vi "Read_Camram_Example.vi"() -> ()   [LabVIEW 2019]
uses:
  camera/Camera.lvclass
  <vilib>/picture/picture.llb/Draw True-Color Pixmap.vi
  <vilib>/picture/picture.llb/Draw 8-Bit Pixmap.vi
panel:
  out "colormap(U8)":u32[](array[numeric])
  out "Image(U16)":u16[][](graph)
  in  "Zoom [%]":i32(slide)=26 min=10 max=200 step=5 scale=10.0..200.0
  out "Image":picture
  out "rawImage":u16[][](array[numeric])
  in  "data_format":T1(ring)=enum."Mono16"
  in  "Image Index":u32 max=1084
  out "Recorded Images":u32
  in  "Quit":bool
  in  "roiY1":u64=2 min=2 max=1440 step=1
  in  "roiX1":u64=2 min=2 max=1920 step=1
  in  "roiY0":u64=1 min=1 max=1439 step=1
  in  "roiX0":u64=1 min=1 max=1919 step=1
  out "Image Height":u16
  out "Image Width":u16
  in  "segment":u16=3 caption="Segment" min=1 max=4
  out "Error":errorcluster {"code" format="%x"}
  # "This example shows for cameras with internal memory how to read images from ram, already available from a previous record\nIt is a good starting point for writing own applications.\nBut it will not be fail save, i.e. doesnt react on errors, just handles them forward to the end\n\nUsage:\nSelect the segment you want to read from before you start the program. \nThis segment must already contain images, otherwise the read will fail\nOnce started, the camera class will be initialized and images will be recorded automatically.\nWhen acquisition has finished you can address the images and set a certain roi \nTo finish the program click on quit application, this will force fan exit of the camera class"
  # "pco.labview"
  # "Camera Setup"
  # "Recording Control"
  # "Parameters for image readout"
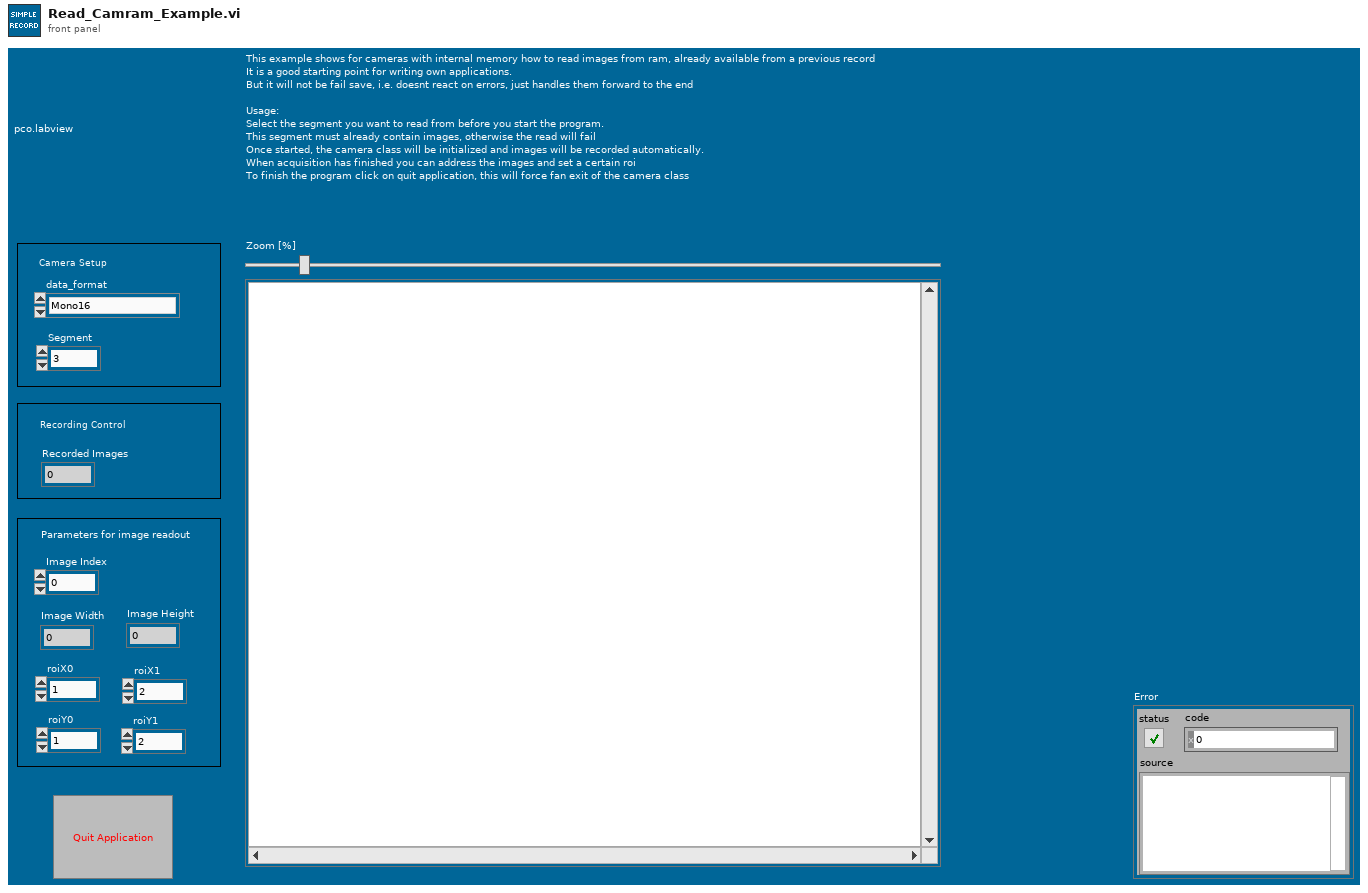
[diagram p1: front panel]
types:
  T1 = enum16{"Undefined", "Mono8", "Mono16", "BGRA8", "RGBA8", "BGRA16", "RGBA16", "CompressedMono8"}
  T2 = enum8{"Enabled", "Disabled", "Disabled and Grayed Out"}
  T3 = typedef "Camera.lvclass/binning.ctl" = cluster{"vert":u16, "horz":u16, "mode":u16}
  T4 = cluster{"exposure_time_s":dbl, "delay_time_s":dbl, "roi":cluster{"x0":u64, "y0":u64, "x1":u64, "y1":u64}, "timestamp_mode":u16, "pixelrate":u32, "conversion_factor":sgl, "trigger_mode":u16, "acquire_mode":u16, "acquire_sequence_number":u32, "metadata_mode":u16, "noisefilter_mode":u16, "pixel_format":u32, "binning":T3, "auto_exposure":cluster{"region":u16, "min_exposure_s":dbl, "max_exposure_s":dbl}}
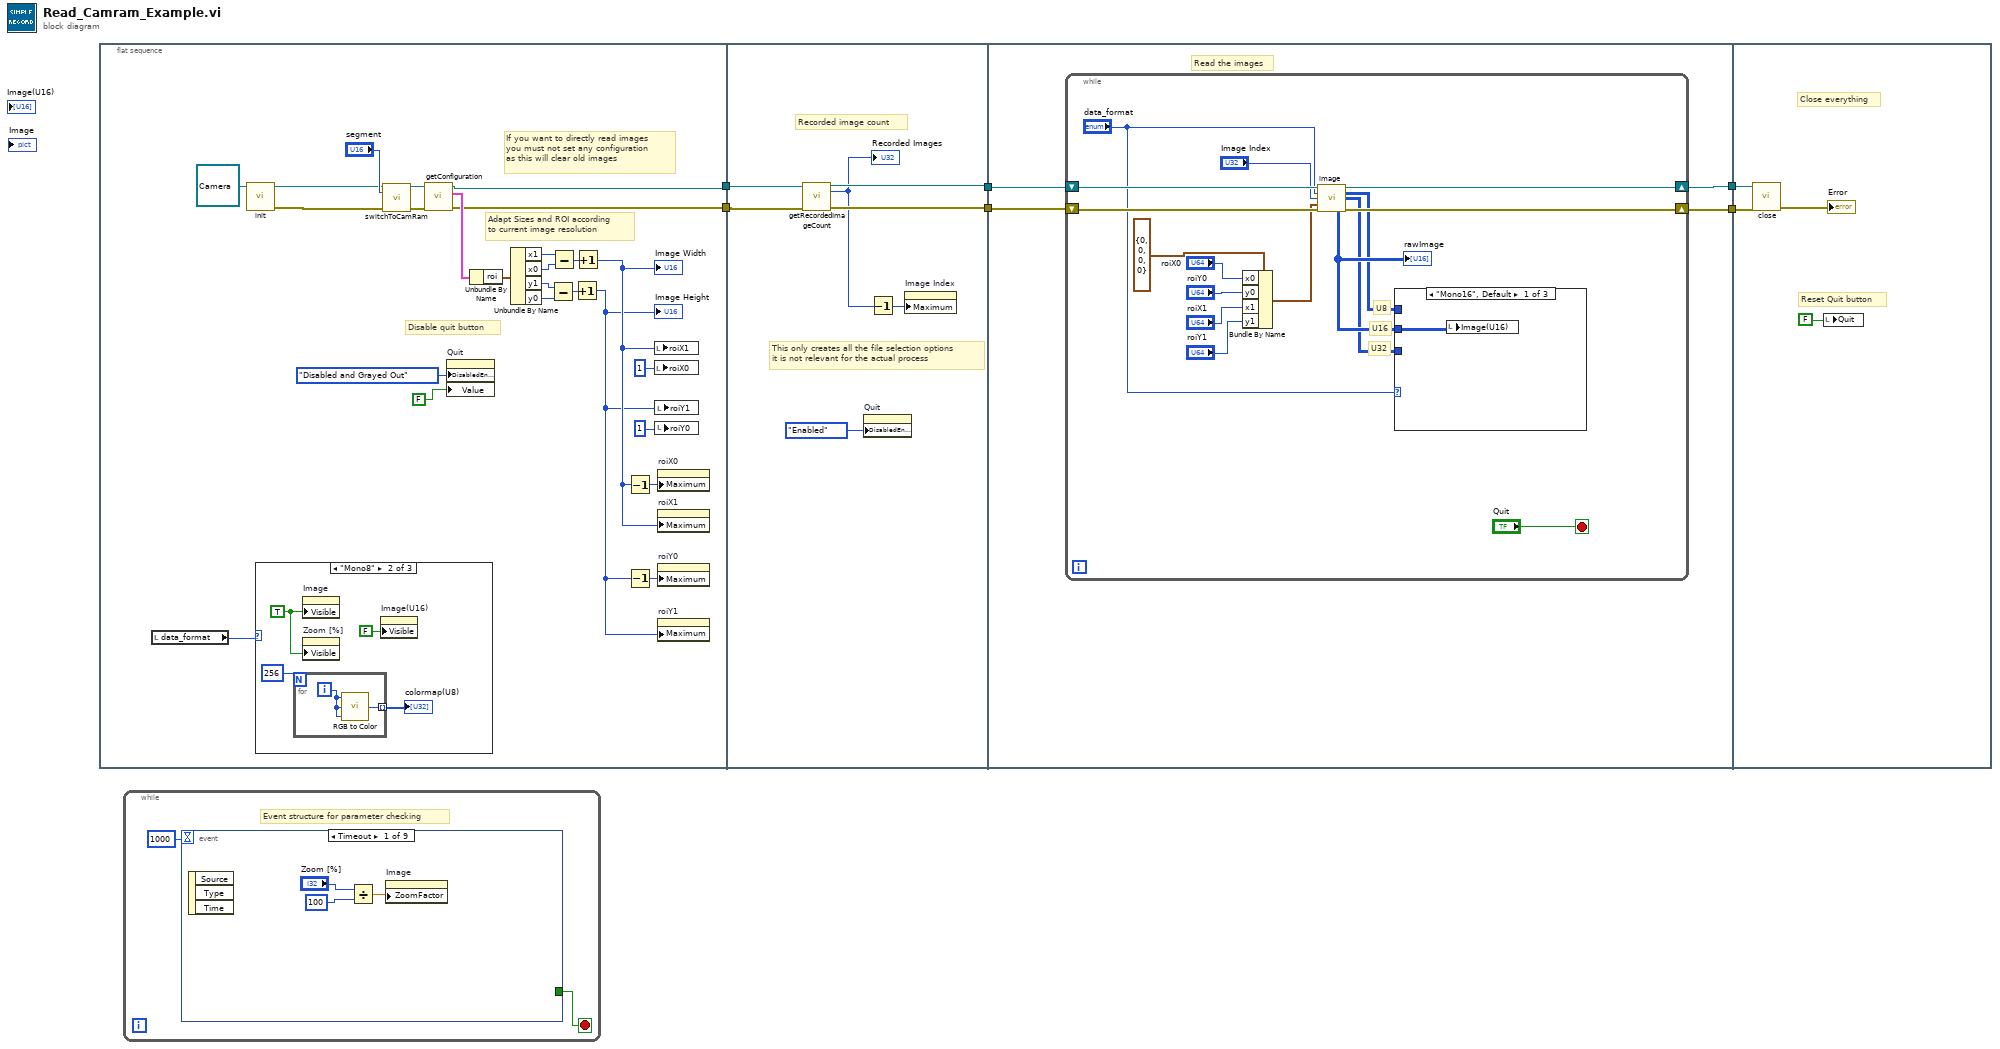
[diagram p0: block diagram]
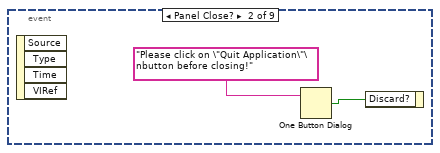
[diagram p2: hidden frame]
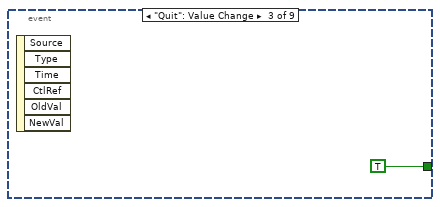
[diagram p3: hidden frame]
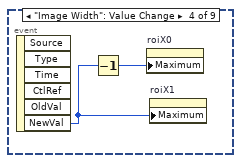
[diagram p4: hidden frame]
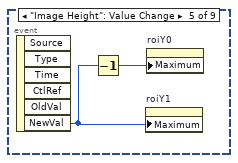
[diagram p5: hidden frame]
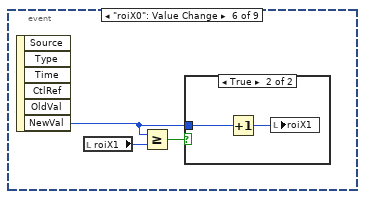
[diagram p6: hidden frame]
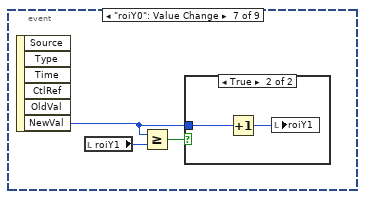
[diagram p8: hidden frame]
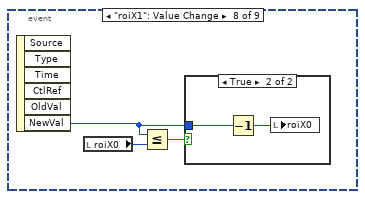
[diagram p10: hidden frame]
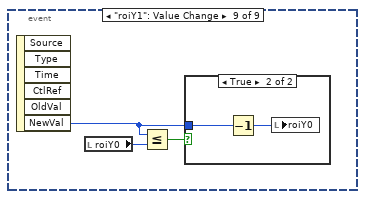
[diagram p12: hidden frame]
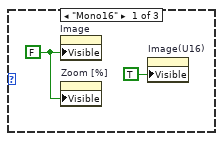
[diagram p14: hidden frame]
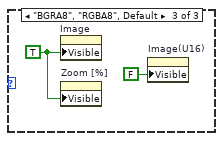
[diagram p15: hidden frame]
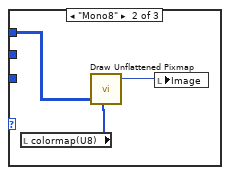
[diagram p16: hidden frame]
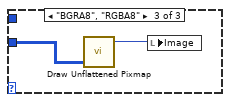
[diagram p17: hidden frame]
diagram:
  n1 = flat-sequence {
    tunnel: [w8] -> w6
    tunnel: [w7] -> w5
    tunnel: [w48] -> w4
    tunnel: [w47] -> w3
    tunnel: w6 -> [w43]
    tunnel: w5 -> [w42]
    tunnel: w4 -> [w51]
    tunnel: w3 -> [w52]
    tunnel: [w50] -> w2
    tunnel: [w49] -> w1
    tunnel: w2 -> [w76]
    tunnel: w1 -> [w75]
    frame #0 {
      # "If you want to directly read images\nyou must not set any configuration\nas this will clear old images"
      # "Adapt Sizes and ROI according\nto current image resolution"
      # "Disable quit button"
      n2 = local read "data_format"() -> (w14:T1)
      n3 = call-dynamic "init.vi"("Camera in"=refnum<class "Camera.lvclass"> refnum ("PCOCamera in")) -> ("Camera out"=w10:refnum<class "Camera.lvclass">, "error out"=w9:errorcluster)  [unwired: 8 in]
      n4 = case shown="\"Mono8\"" w14 {
        frame "Mono16" {
          w33 = FALSE ("Visible")
          n5 = property on="Image" class="Pict"("Visible"=w33) -> ()  [unwired: 2 in, 2 out]
          n6 = property on="Zoom [%]" class="Slide (strict)"("Visible"=w33) -> ()  [unwired: 2 in, 2 out]
          n7 = property on="Image(U16)" class="IntGraph (strict)"("Visible"=TRUE) -> ()  [unwired: 2 in, 2 out]
        }
        frame "Mono8" {
          w36 = TRUE ("Visible")
          n8 = for {
            N: 256 -> [_]
            tunnel: [w38] -> w35 mode=indexing
            i -> [w39]
            n9 = call <vilib>:"RGB to Color.vi"("B"=w39, "G"=w39, "R"=w39) -> ("Color"=w38:u32)
          }
          "colormap(U8)" <- w35
          n10 = property on="Image" class="Pict"("Visible"=w36) -> ()  [unwired: 2 in, 2 out]
          n11 = property on="Zoom [%]" class="Slide (strict)"("Visible"=w36) -> ()  [unwired: 2 in, 2 out]
          n12 = property on="Image(U16)" class="IntGraph (strict)"("Visible"=FALSE) -> ()  [unwired: 2 in, 2 out]
        }
        frame "BGRA8", "RGBA8", Default {
          w40 = TRUE ("Visible")
          n13 = property on="Image" class="Pict"("Visible"=w40) -> ()  [unwired: 2 in, 2 out]
          n14 = property on="Zoom [%]" class="Slide (strict)"("Visible"=w40) -> ()  [unwired: 2 in, 2 out]
          n15 = property on="Image(U16)" class="IntGraph (strict)"("Visible"=FALSE) -> ()  [unwired: 2 in, 2 out]
        }
      }
      n16 = call-dynamic "switchToCamRam.vi"("Camera in"=w10, "segment"="segment", "error in (no error)"=w9) -> ("Camera out"=w12:refnum<class "Camera.lvclass">, "error out"=w11:errorcluster)  [unwired: 11 in]
      n17 = call-dynamic "getConfiguration.vi"("error in (no error)"=w11, "Camera in"=w12) -> ("error out"=w7:errorcluster, "configuration"=w26:T4, "Camera out"=w8:refnum<class "Camera.lvclass">)  [unwired: 7 in]
      n18 = property on="Quit" class="Bool (strict)"("DisabledEnum"=T2."Disabled and Grayed Out" ("Disabled"), "Value"=FALSE ("Stop")) -> ()  [unwired: 2 in, 2 out]
      n19 = Unbundle By Name(w26) -> ("roi"=w25:cluster{"x0":u64, "y0":u64, "x1":u64, "y1":u64})
      n20 = Unbundle By Name(w25) -> ("x1"=w23:u64, "x0"=w24:u64, "y1"=w21:u64, "y0"=w22:u64)
      n21 = Subtract(x=w21, y=w22) -> (x-y=w19:u64)
      n22 = Subtract(x=w23, y=w24) -> (x-y=w20:u64)
      n23 = Increment(x=w19) -> (x+1=w17:u64)
      "Image Height" <- w17
      n24 = Increment(x=w20) -> (x+1=w18:u64)
      "Image Width" <- w18
      n25 = Decrement(x=w18) -> (x-1=w28:u64)
      n26 = Decrement(x=w17) -> (x-1=w27:u64)
      n27 = local write "roiX1"(w18) -> ()
      n28 = local write "roiX0"(u16 1 ("roiY0")) -> ()
      n29 = local write "roiY1"(w17) -> ()
      n30 = local write "roiY0"(u16 1 ("roiY0")) -> ()
      n31 = property on="roiX0" class="DigNum (strict)"("Maximum"=w28) -> ()  [unwired: 2 in, 2 out]
      n32 = property on="roiX1" class="DigNum (strict)"("Maximum"=w18) -> ()  [unwired: 2 in, 2 out]
      n33 = property on="roiY0" class="DigNum (strict)"("Maximum"=w27) -> ()  [unwired: 2 in, 2 out]
      n34 = property on="roiY1" class="DigNum (strict)"("Maximum"=w17) -> ()  [unwired: 2 in, 2 out]
    }
    frame #1 {
      # "This only creates all the file selection options\nit is not relevant for the actual process"
      # "Recorded image count"
      n35 = call-dynamic "getRecordedImageCount.vi"("Camera in"=w43, "error in (no error)"=w42) -> ("Camera out"=w48:refnum<class "Camera.lvclass">, "recorded_image_count"=w44:u32, "error out"=w47:errorcluster)  [unwired: 11 in]
      "Recorded Images" <- w44
      n36 = property on="Quit" class="Bool (strict)"("DisabledEnum"=T2."Enabled" ("Disabled")) -> ()  [unwired: 2 in, 2 out]
      n37 = Decrement(x=w44) -> (x-1=w45:u32)
      n38 = property on="Image Index" class="DigNum (strict)"("Maximum"=w45) -> ()  [unwired: 2 in, 2 out]
    }
    frame #2 {
      # "Read the images"
      n39 = while {
        shift-right: [w66] -> w50
        shift-left: w51 -> [w68]
        shift-right: [w61] -> w49
        shift-left: w52 -> [w67]
        stop <- "Quit" stop-if-true
        # "U32"
        # "U16"
        # "U8"
        n40 = Bundle By Name(cluster=cluster{"x0":u64, "y0":u64, "x1":u64, "y1":u64} {"x0"=0, "y0"=0, "x1"=0, "y1"=0} ("roi"), "x0"="roiX0", "y0"="roiY0", "x1"="roiX1", "y1"="roiY1") -> (w60:cluster{"x0":u64, "y0":u64, "x1":u64, "y1":u64})
        n41 = call-dynamic "image.vi"("Camera in"=w68, "data_format"="data_format", "image_index"="Image Index", "crop"=w60, "error in (no error)"=w67) -> ("Camera out"=w66:refnum<class "Camera.lvclass">, "image (U8)"=w53:u8[][], "image (U32)"=w54:u32[][], "raw_image (U16)"=w55:u16[][], "error out"=w61:errorcluster)  [unwired: 2 in, 4 out]
        "rawImage" <- w55
        n42 = case shown="\"Mono16\", Default" "data_format" {
          tunnel: w54 -> [_ _ w74]
          tunnel: w53 -> [_ w71 _]
          tunnel: w55 -> [w69 _ _]
          frame "Mono16", Default {
            n43 = local write "Image(U16)"(w69) -> ()
          }
          frame "Mono8" {
            n44 = local read "colormap(U8)"() -> (w70:u32[])
            n45 = call-poly <vilib>:"Draw Unflattened Pixmap.vi"("data"=w71, "color table"=w70) -> ("new picture"=w72:picture)  [unwired: 7 in]
            n46 = local write "Image"(w72) -> ()
          }
          frame "BGRA8", "RGBA8" {
            n47 = call-poly <vilib>:"Draw Unflattened Pixmap.vi"("data (RGB format)"=w74) -> ("new picture"=w73:picture)  [unwired: 8 in]
            n48 = local write "Image"(w73) -> ()
          }
        }
      }
    }
    frame #3 {
      # "Reset Quit button"
      # "Close everything"
      n49 = call-dynamic "close.vi"("error in (no error)"=w75, "Camera in"=w76) -> ("error out"=→"Error":errorcluster)  [unwired: 9 in]
      n50 = local write "Quit"(FALSE ("Stop")) -> ()
    }
  }
  n51 = while {
    stop <- w79 stop-if-true
    # "Event structure for parameter checking"
    n52 = event shown="[0] Timeout" {
      selector: _ -> [_ _ _ _ _ _ _ _ _]
      dyn-events: _ -> [_ _ _ _ _ _ _ _ _]
      timeout: 1000 -> [_ _ _ _ _ _ _ _ _]
      tunnel: [_ _ TRUE _ _ _ _ _ _] -> w79
      event Timeout {
        n53 = event-data() -> ()  [unwired: 1 in, 3 out]
        n54 = Divide(x="Zoom [%]", y=100 ("Zoom [%]")) -> (x/y=w81:dbl)
        n55 = property on="Image" class="Pict"("ZoomFactor"=w81) -> ()  [unwired: 2 in, 2 out]
      }
      event Panel Close? {
        n56 = event-data() -> ()  [unwired: 1 in, 4 out]
        n57 = One Button Dialog(message="Please click on \"Quit Application\"\nbutton before closing!") -> (true=w84:bool)  [unwired: 1 in]
        n58 = event-data("Discard?"=w84) -> ()  [unwired: 1 in, 1 out]
      }
      event "Quit": Value Change {
        n59 = event-data() -> ()  [unwired: 1 in, 6 out]
      }
      event "Image Width": Value Change {
        n60 = event-data() -> ("NewVal"=w87:u16)  [unwired: 1 in, 5 out]
        n61 = Decrement(x=w87) -> (x-1=w88:u16)
        n62 = property on="roiX0" class="DigNum (strict)"("Maximum"=w88) -> ()  [unwired: 2 in, 2 out]
        n63 = property on="roiX1" class="DigNum (strict)"("Maximum"=w87) -> ()  [unwired: 2 in, 2 out]
      }
      event "Image Height": Value Change {
        n64 = event-data() -> ("NewVal"=w89:u16)  [unwired: 1 in, 5 out]
        n65 = Decrement(x=w89) -> (x-1=w90:u16)
        n66 = property on="roiY1" class="DigNum (strict)"("Maximum"=w89) -> ()  [unwired: 2 in, 2 out]
        n67 = property on="roiY0" class="DigNum (strict)"("Maximum"=w90) -> ()  [unwired: 2 in, 2 out]
      }
      event "roiX0": Value Change {
        n68 = event-data() -> ("NewVal"=w91:u64)  [unwired: 1 in, 5 out]
        n69 = local read "roiX1"() -> (w93:u64)
        n70 = Greater Or Equal?(x=w91, y=w93) -> (x >= y?=w92:bool)
        n71 = case shown="True" w92 {
          tunnel: w91 -> [_ w95]
          frame False {
          }
          frame True {
            n72 = Increment(x=w95) -> (x+1=w94:u64)
            n73 = local write "roiX1"(w94) -> ()
          }
        }
      }
      event "roiY0": Value Change {
        n74 = event-data() -> ("NewVal"=w96:u64)  [unwired: 1 in, 5 out]
        n75 = local read "roiY1"() -> (w98:u64)
        n76 = Greater Or Equal?(x=w96, y=w98) -> (x >= y?=w97:bool)
        n77 = case shown="True" w97 {
          tunnel: w96 -> [_ w100]
          frame False {
          }
          frame True {
            n78 = Increment(x=w100) -> (x+1=w99:u64)
            n79 = local write "roiY1"(w99) -> ()
          }
        }
      }
      event "roiX1": Value Change {
        n80 = event-data() -> ("NewVal"=w101:u64)  [unwired: 1 in, 5 out]
        n81 = local read "roiX0"() -> (w103:u64)
        n82 = Less Or Equal?(x=w101, y=w103) -> (x <= y?=w102:bool)
        n83 = case shown="True" w102 {
          tunnel: w101 -> [_ w105]
          frame False {
          }
          frame True {
            n84 = Decrement(x=w105) -> (x-1=w104:u64)
            n85 = local write "roiX0"(w104) -> ()
          }
        }
      }
      event "roiY1": Value Change {
        n86 = event-data() -> ("NewVal"=w106:u64)  [unwired: 1 in, 5 out]
        n87 = local read "roiY0"() -> (w108:u64)
        n88 = Less Or Equal?(x=w106, y=w108) -> (x <= y?=w107:bool)
        n89 = case shown="True" w107 {
          tunnel: w106 -> [_ w110]
          frame False {
          }
          frame True {
            n90 = Decrement(x=w110) -> (x-1=w109:u64)
            n91 = local write "roiY0"(w109) -> ()
          }
        }
      }
    }
  }
